vi "REPL_Comm.vi"(8 "REPL Name":string="Robot  REPL", 9 "CodeRef":refnum<vi>, 11 "Microprocessor in":T2) -> (3 "Microprocessor out":T2)   [LabVIEW 2016]
uses:
  uPythonX/uPythonX.xctl
  ColorText/Code.xctl
  <vilib>/Utility/miscctls.llb/LVPointTypeDef.ctl
panel:
  out "mouse down?":bool
  in  "VISA":refnum<visa-resource-name>
  out "Old Code":string
  in  "Files":u16(ring) items=["README.txt", "Screen.py", "boot.py", "fwupdate.mpy", "pybcdc.inf", "main.py"]
  in  "Ctrls":T1(ring)
  in  "HelpCode":string
  in  "Stop Script":bool
  in  "Pause":bool
  in  "Help Button":bool
  in  "New":bool
  in  "Delete":bool
  in  "refresh":bool
  in  "Code":string(xcontrol)="import utime\n\nfor i in range(5):\n     led.value(0)\n     utime.sleep_ms(1000)\n     led.value(1)\n     utime.sleep_ms(1000)\n\n\n\nprint('hi')"
  out "Script":string
  in  "Copy":bool
  out "String":string
  in  "Clear":bool
  out "Origin":T3
  in  "Ctrl D":bool
  in  "Ctrl C":bool
  in  "Run DIrect":bool
  in  "Run":bool
  out "Console":string
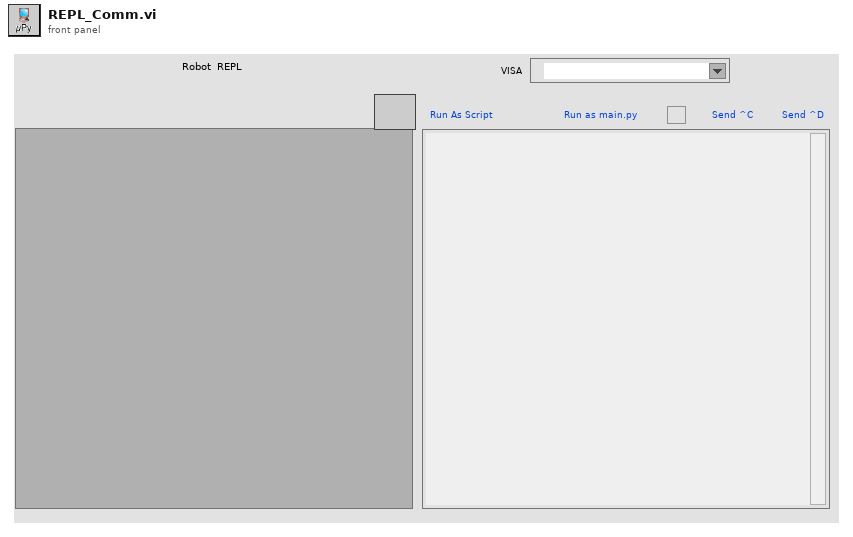
[diagram p1: front panel]
types:
  T1 = enum16{"File Control", "Save to PC", "Read from PC", "Save to MP as..."}
  T2 = cluster{"VISA Refnum in":refnum<visa-resource-name>, "Python Code":string}
  T3 = typedef "LVPointTypeDef.ctl" = cluster{"Horizontal":i16, "Vertical":i16}
  T4 = cluster{"VISA out":refnum<visa-resource-name>, "Code":string}
  T5 = typedef "eventvkey.ctl" = enum16{"ASCII", "Enter", "Return", "Shift", "Ctrl", "Alt", "Cmd", "Opt", "Caps", "NumLock", "Clear", "Break", "Up", "Down", "Left", "Right", "Insert", "Delete", "Home", "End", "PageUp", "PageDown", "Escape", "Help", "Pause", "ScrollLock", "F1", "F2", "F3", "F4", "F5", "F6", "F7", "F8", "F9", "F10", "F11", "F12", "F13", "F14", "F15", "F16", "F17", "F18", "F19", "F20", "F21", "F22", "F23", "F24", "Play", "VolumeUp", "VolumeDown", "Mute", "Two Byte Char"}
  T6 = cluster{"Shift":bool, "Ctrl":bool, "Alt":bool, "Cmd":bool, "Opt":bool}
  T7 = cluster{"Char":i16, "VKey":T5, "ScanCode":i16, "Mods":cluster{"Num Pad":bool, "Menu Key":bool}, "PlatMods":cluster{"Shift":bool, "Ctrl":bool, "Alt":bool, "Cmd":bool, "Opt":bool}, "FocusObj":refnum<vi>}
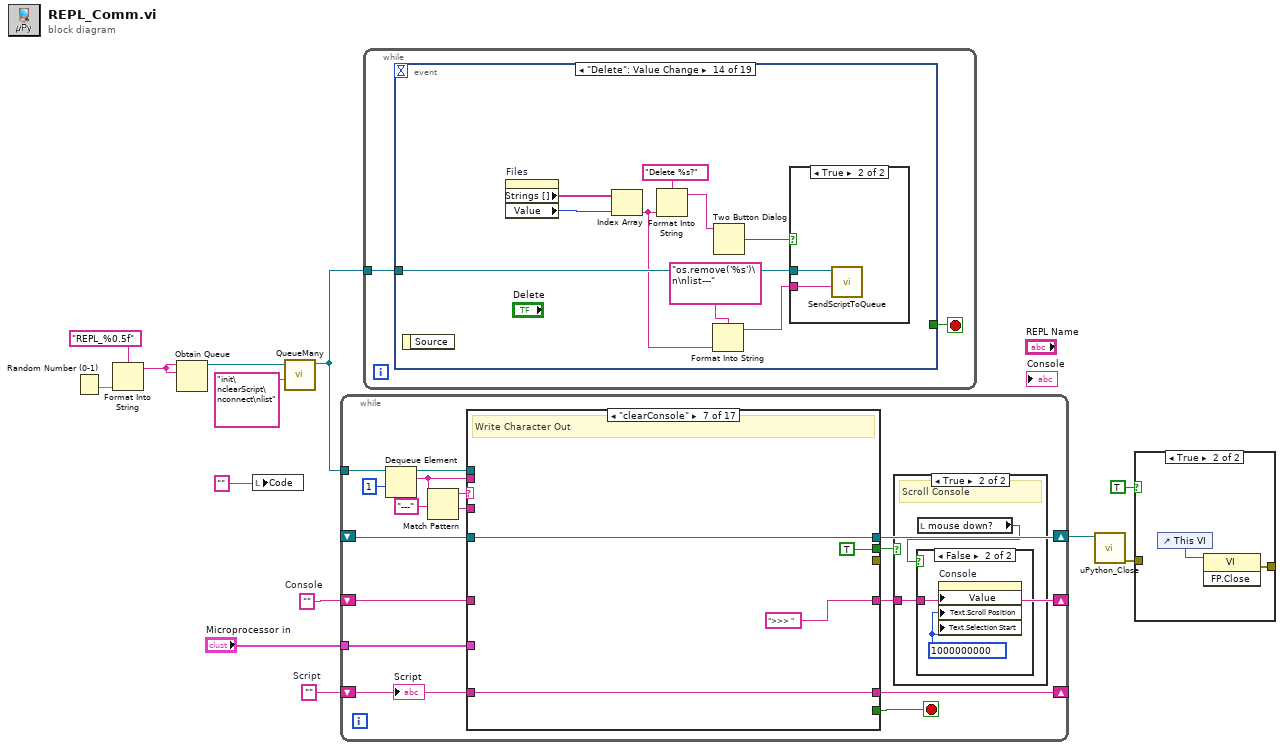
[diagram p0: block diagram]
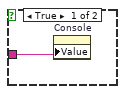
[diagram p4: hidden frame]
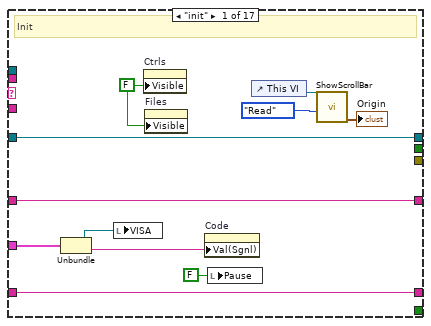
[diagram p5: hidden frame]
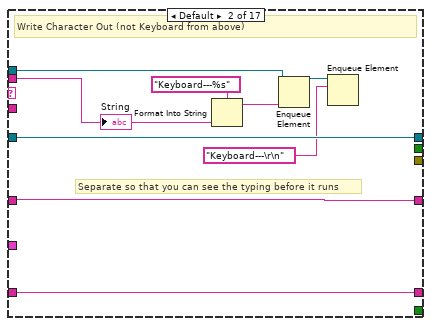
[diagram p6: hidden frame]
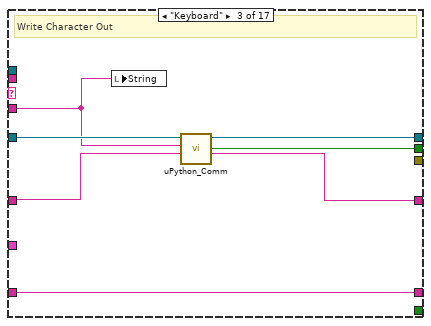
[diagram p7: hidden frame]
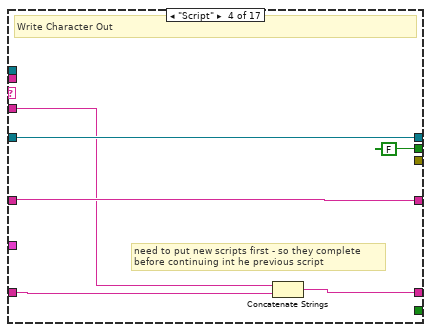
[diagram p8: hidden frame]
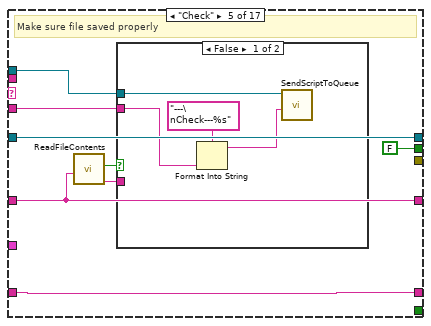
[diagram p9: hidden frame]
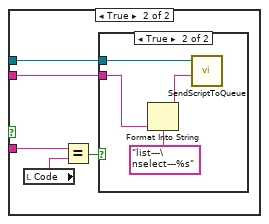
[diagram p10: hidden frame]
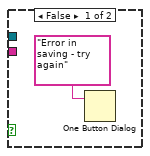
[diagram p11: hidden frame]
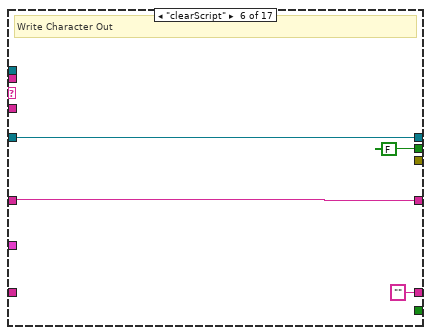
[diagram p12: hidden frame]
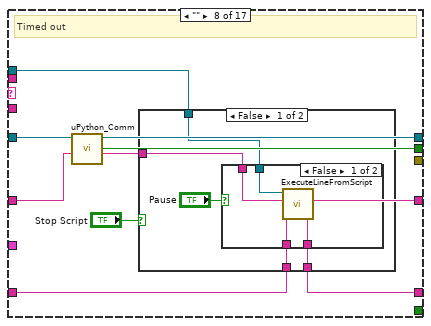
[diagram p13: hidden frame]
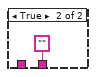
[diagram p15: hidden frame]
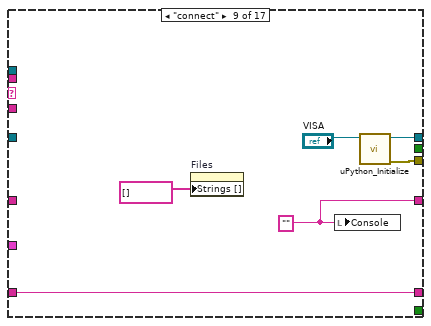
[diagram p16: hidden frame]
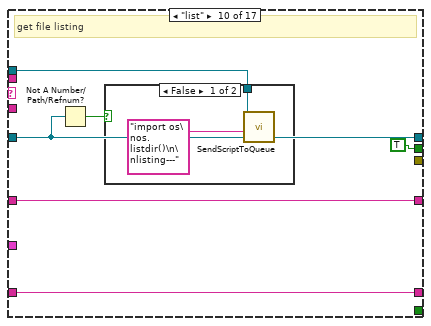
[diagram p17: hidden frame]
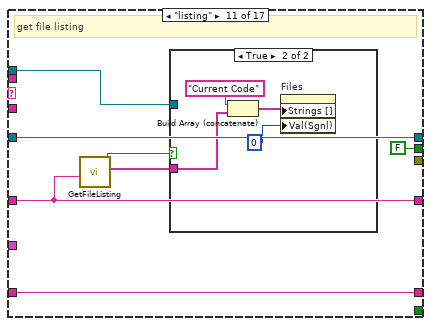
[diagram p19: hidden frame]
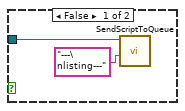
[diagram p20: hidden frame]
diagram:
  w8 = ""  # Script
  w9 = ""  # Console
  n1 = Random Number (0-1)() -> (number: 0 to 1=w2:dbl)
  n2 = Format Into String(format string="REPL_%0.5f" ("name (unnamed)"), w2) -> (resulting string=w1:string)  [unwired: 2 in, 1 out]
  n3 = Obtain Queue(name (unnamed)=w1, element data type=w1) -> (queue out=w13:refnum<queue>)  [unwired: 3 in, 2 out]
  n4 = local write "Code"("" ("Code")) -> ()
  n5 = call "QueueMany.vi"("Playlist"="init\nclearScript\nconnect\nlist" ("element"), "Queue in"=w13) -> ("Queue out"=w12:refnum<queue>)  [unwired: 9 in]
  n6 = while {
    tunnel: w12 -> [w29]
    shift-right: [w19] -> w10
    shift-left: _ -> [w27]
    shift-right: [w18] -> _
    shift-left: w9 -> [w20]
    shift-right: [w16] -> _
    shift-left: w8 -> [w15]
    tunnel: "Microprocessor in" -> [w14]
    stop <- w28 stop-if-true
    n7 = Dequeue Element(queue=w29, timeout in ms (-1)=1) -> (queue out=w25:refnum<queue>, element=w21:string)  [unwired: 1 in, 2 out]
    n8 = Match Pattern(string=w21, regular expression="---") -> (before substring=w23:string, after substring=w22:string)  [unwired: 1 in, 2 out]
    n9 = case shown="\"clearConsole\"" w23 {
      tunnel: [_ _ _ _ _ _ _ _ _ _ _ _ _ _ _ _ TRUE] -> w28
      tunnel: w27 -> [w45 w53 w60 w67 w75 w93 w97 w103 _ w125 w135 w148 w153 w173 w179 w185 w196]
      tunnel: w25 -> [_ w46 _ _ w71 _ _ w106 _ w127 w132 w145 _ _ _ _ _]
      tunnel: w22 -> [_ _ w55 w62 w68 _ _ _ _ _ _ _ _ w174 _ _ _]
      tunnel: w21 -> [_ w48 _ _ _ _ _ _ _ _ _ _ _ _ _ _ _]
      tunnel: [w45 w53 w58 w67 w75 w93 w97 w100 w123 w125 w135 w148 w161 w173 w179 w185 w196] -> w19
      tunnel: w20 -> [w44 w52 w59 w66 w70 w92 _ w102 _ w126 w134 w147 w156 w172 w182 w187 w197]
      tunnel: [w44 w52 w57 w66 w70 w92 ">>> " ("Console") w101 w121 w126 w134 w147 w159 w172 w182 w187 w197] -> w18
      tunnel: [_ _ _ _ _ _ _ _ w122 _ _ _ w158 _ _ _ _] -> _
      tunnel: [_ _ w56 FALSE ("Update?") FALSE ("Update?") FALSE ("Update?") TRUE ("Update?") w99 _ TRUE ("Update?") FALSE ("Update?") _ _ _ _ _ _] -> w17
      tunnel: [w42 w54 w61 w64 w73 "" ("Script") w95 w105 w119 w128 w136 w150 w167 w171 w181 w186 w194] -> w16
      tunnel: w15 -> [w42 w54 w61 w63 w73 _ w95 w104 w119 w128 w136 w150 w167 w171 w181 w186 w194]
      tunnel: w14 -> [w41 _ _ _ _ _ _ _ _ _ _ _ _ _ _ _ w192]
      frame "init" {
        w38 = FALSE ("Visible")
        # "Init"
        n10 = Unbundle(w41) -> ("VISA Refnum in"=w43:refnum<visa-resource-name>, "Python Code"=w40:string)
        n11 = local write "VISA"(w43) -> ()
        n12 = property on="Ctrls" class="Enum (strict)"("Visible"=w38) -> ()  [unwired: 2 in, 2 out]
        n13 = property on="Files" class="Ring (strict)"("Visible"=w38) -> ()  [unwired: 2 in, 2 out]
        n14 = property on="Code" class="Code (strict)"("Val(Sgnl)"=w40) -> ()  [unwired: 2 in, 2 out]
        n15 = local write "Pause"(FALSE ("Pause")) -> ()
        n16 = control-ref of="This VI"() -> (w37:refnum<vi>)
        n17 = call "ShowScrollBar.vi"("Task"=enum16{"Read", "Change", "Reset"}."Read", "VI in"=w37) -> ("Origin"=→"Origin":T3)  [unwired: 9 in]
      }
      frame Default {
        # "Separate so that you can see the typing before it runs"
        # "Write Character Out (not Keyboard from above)"
        n18 = Format Into String(format string="Keyboard---%s", w48) -> (resulting string=w50:string)  [unwired: 2 in, 1 out]
        n19 = Enqueue Element(queue=w46, element=w50) -> (queue out=w49:refnum<queue>)  [unwired: 2 in, 2 out]
        n20 = Enqueue Element(queue=w49, element="Keyboard---\r\n" ("regular expression")) -> ()  [unwired: 2 in, 3 out]
        "String" <- w48
      }
      frame "Keyboard" {
        # "Write Character Out"
        n21 = local write "String"(w55) -> ()
        n22 = call "uPython_Comm.vi"("Console In"=w59, "Script"=w55, "VISA Refnum in"=w60) -> ("Console Out"=w57:string, "VISA out"=w58:refnum<visa-resource-name>, "Update?"=w56:bool)  [unwired: 4 in, 2 out]
      }
      frame "Script" {
        # "need to put new scripts first - so they complete\nbefore continuing int he previous script"
        # "Write Character Out"
        n23 = Concatenate Strings(w62, w63) -> (w64:string)
      }
      frame "Check" {
        # "Make sure file saved properly"
        n24 = call "ReadFileContents.vi"("Console"=w70) -> ("File Contents"=w69:string, "Success?"=w72:bool)  [unwired: 9 in]
        n25 = case shown="False" w72 {
          tunnel: w71 -> [w79 w80]
          tunnel: w69 -> [_ w83]
          tunnel: w68 -> [w77 w82]
          frame False {
            n26 = Format Into String(format string="---\nCheck---%s" ("String"), w77) -> (resulting string=w76:string)  [unwired: 2 in, 1 out]
            n27 = call "SendScriptToQueue.vi"("String"=w76, "Queue in"=w79) -> ()  [unwired: 10 in]
          }
          frame True {
            n28 = local read "Code"() -> (w84:string)
            n29 = Equal?(x=w83, y=w84) -> (x = y?=w81:bool)
            n30 = case shown="True" w81 {
              tunnel: w82 -> [_ w88]
              tunnel: w80 -> [_ w87]
              frame False {
                n31 = One Button Dialog(message="Error in saving - try again" ("Code")) -> ()  [unwired: 1 in, 1 out]
              }
              frame True {
                n32 = Format Into String(format string="list---\nselect---%s" ("element"), w88) -> (resulting string=w86:string)  [unwired: 2 in, 1 out]
                n33 = call "SendScriptToQueue.vi"("String"=w86, "Queue in"=w87) -> ()  [unwired: 10 in]
              }
            }
          }
        }
      }
      frame "clearScript" {
        # "Write Character Out"
      }
      frame "clearConsole" {
        # "Write Character Out"
      }
      frame "" {
        # "Timed out"
        n34 = call "uPython_Comm.vi"("Console In"=w102, "VISA Refnum in"=w103) -> ("Console Out"=w101:string, "VISA out"=w100:refnum<visa-resource-name>, "Update?"=w99:bool)  [unwired: 5 in, 2 out]
        n35 = case shown="False" "Stop Script" {
          tunnel: w106 -> [w111 _]
          tunnel: [w110 "" ("Script")] -> w105
          tunnel: w104 -> [w109 _]
          tunnel: w101 -> [w108 _]
          frame False {
            n36 = case shown="False" "Pause" {
              tunnel: w111 -> [w115 _]
              tunnel: [w114 w116] -> w110
              tunnel: w109 -> [w113 w116]
              tunnel: w108 -> [w112 _]
              frame False {
                n37 = call "ExecuteLineFromScript.vi"("Script in"=w113, "Console"=w112, "Queue in"=w115) -> ("Script out"=w114:string)  [unwired: 8 in]
              }
              frame True {
              }
            }
          }
          frame True {
          }
        }
      }
      frame "connect" {
        w121 = "" ("element")
        n38 = property on="Files" class="Ring (strict)"("Strings []"=string[] [] ("Item Names")) -> ()  [unwired: 2 in, 2 out]
        n39 = local write "Console"(w121) -> ()
        n40 = call "uPython_Initialize.vi"("VISA Refnum in"="VISA") -> ("error out"=w122:errorcluster, "VISA Refnum out"=w123:refnum<visa-resource-name>)  [unwired: 9 in]
      }
      frame "list" {
        # "get file listing"
        n41 = Not A Number/Path/Refnum?(number/path/refnum=w125) -> (NaN/Path/Refnum?=w124:bool)
        n42 = case shown="False" w124 {
          tunnel: w127 -> [w131 _]
          frame False {
            n43 = call "SendScriptToQueue.vi"("String"="import os\nos.listdir()\n\nlisting---" ("element"), "Queue in"=w131) -> ()  [unwired: 10 in]
          }
          frame True {
          }
        }
      }
      frame "listing" {
        # "get file listing"
        n44 = call "GetFileListing.vi"("Console In"=w134) -> ("Files"=w138:string[], "Success?"=w133:bool)  [unwired: 9 in]
        n45 = case shown="True" w133 {
          tunnel: w138 -> [_ w144]
          tunnel: w132 -> [w139 _]
          frame False {
            n46 = call "SendScriptToQueue.vi"("String"="---\nlisting---", "Queue in"=w139) -> ()  [unwired: 10 in]
          }
          frame True {
            n47 = Build Array (concatenate)("Current Code", w144) -> (w143:string[])
            n48 = property on="Files" class="Ring (strict)"("Strings []"=w143, "Val(Sgnl)"=0) -> ()  [unwired: 2 in, 2 out]
          }
        }
      }
      frame "read" {
        n49 = call "ReadFileContents.vi"("Console"=w147) -> ("File Contents"=w149:string, "Success?"=w146:bool)  [unwired: 9 in]
        n50 = local write "Code"(w149) -> ()
        n51 = case shown="False" w146 {
          tunnel: w145 -> [w152 _]
          frame False {
            n52 = call "SendScriptToQueue.vi"("String"="---\nread---", "Queue in"=w152) -> ()  [unwired: 10 in]
          }
          frame True {
          }
        }
      }
      frame "run" {
        w157 = "\u0003"  # Ctrl C
        w164 = "\u0004"  # Ctrl D
        # "run on main.py"
        n53 = call "uPython_Comm.vi"("Console In"=w156, "Script"=w157, "VISA Refnum in"=w153) -> ("error out"=w155:errorcluster, "VISA out"=w154:refnum<visa-resource-name>)  [unwired: 4 in, 3 out]
        n54 = local read "Code"() -> (w160:string)
        n55 = call "SavePyFile.vi"("Name"="main.py", "error in"=w155, "Python Code"=w160, "VISA in"=w154) -> ("error out"=w165:errorcluster, "Reply"=w163:string, "VISA out"=w166:refnum<visa-resource-name>)  [unwired: 5 in]
        n56 = call "uPython_Comm.vi"("error in (no error)"=w165, "Console In"=w163, "Script"=w164, "VISA Refnum in"=w166) -> ("error out"=w158:errorcluster, "Console Out"=w159:string, "VISA out"=w161:refnum<visa-resource-name>)  [unwired: 3 in, 2 out]
      }
      frame "select" {
        n57 = property on="Files" class="Ring (strict)"() -> ("Strings []"=w168:string[])  [unwired: 2 in, 2 out]
        n58 = call <vilib>:"Trim Whitespace.vi"("string"=w174) -> ("trimmed string"=w170:string)  [unwired: 1 in]
        n59 = Search 1D Array(1D array=w168, element=w170) -> (index of element=w169:i32)  [unwired: 1 in]
        n60 = case shown="Default" w169 {
          selector: w169 -> [_ w175]
          frame -1 {
          }
          frame Default {
            n61 = property on="Files" class="Ring (strict)"("Val(Sgnl)"=w175) -> ()  [unwired: 2 in, 2 out]
          }
        }
      }
      frame "help" {
        n62 = local read "Code"() -> (w180:string)
        n63 = control-ref of="HelpCode"() -> (w176:refnum<vi>)
        n64 = Bundle("VISA out"=w179, "Code"=w180) -> (w178:T4)  [unwired: 1 in]
        n65 = call "OpenHelp.vi"("Code Ref"=w176, "Microprocessor in"=w178, "Dialog"=enum16{"REPL", "Help"}."Help") -> ()  [unwired: 9 in]
      }
      frame "update" {
        n66 = local read "Code"() -> (w183:string)
        n67 = property class="Str"(reference="CodeRef", "Val(Sgnl)"=w183) -> ()  [unwired: 1 in, 2 out]
      }
      frame "done" {
        w191 = FALSE ("Visible")
        n68 = local read "Code"() -> (w193:string)
        n69 = property on="Ctrls" class="Enum (strict)"("Visible"=w191) -> ()  [unwired: 2 in, 2 out]
        n70 = Bundle(cluster=w192, "VISA Refnum in"=w196, "Python Code"=w193) -> (→"Microprocessor out":T2)
        n71 = property on="Files" class="Ring (strict)"("Visible"=w191) -> ()  [unwired: 2 in, 2 out]
        n72 = control-ref of="This VI"() -> (w189:refnum<vi>)
        n73 = local read "Origin"() -> (w190:T3)
        n74 = call "ShowScrollBar.vi"("Origin in"=w190, "Task"=enum16{"Read", "Change", "Reset"}."Reset", "VI in"=w189) -> ()  [unwired: 8 in, 1 out]
      }
    }
    n75 = case shown="True" w17 {
      tunnel: w18 -> [_ w31]
      frame False {
      }
      frame True {
        # "Scroll Console"
        n76 = local read "mouse down?"() -> (w30:bool)
        n77 = case shown="False" w30 {
          tunnel: w31 -> [w32 w33]
          frame True {
            n78 = property on="Console" class="Str"("Value"=w32) -> ()  [unwired: 2 in, 2 out]
          }
          frame False {
            w34 = u32 1000000000 ("Text.Selection:Start")
            n79 = property on="Console" class="Str"("Value"=w33, "Text.Scroll Position"=w34, "Text.Selection Start"=w34) -> ()  [unwired: 2 in, 2 out]
          }
        }
      }
    }
    "Script" <- w15
  }
  n80 = while {
    tunnel: w12 -> [w199]
    stop <- w200 stop-if-true
    n81 = event shown="[13] \"Delete\": Value Change" {
      selector: _ -> [_ _ _ _ _ _ _ _ _ _ _ _ _ _ _ _ _ _ _]
      dyn-events: _ -> [_ _ _ _ _ _ _ _ _ _ _ _ _ _ _ _ _ _ _]
      timeout: _ -> [_ _ _ _ _ _ _ _ _ _ _ _ _ _ _ _ _ _ _]
      tunnel: w199 -> [w202 _ _ _ w212 w225 w249 w258 w262 w285 w289 w291 w292 w299 w306 w307 w309 _ w312]
      tunnel: [_ _ _ _ TRUE ("Discard?") _ _ _ _ _ _ _ _ _ _ _ _ _ _] -> w200
      event "Copy": Value Change {
        n82 = event-data() -> ()  [unwired: 1 in, 1 out]
        n83 = call "QueueMany.vi"("Playlist"="update" ("element"), "Queue in"=w202) -> ()  [unwired: 9 in, 1 out]
      }
      event Timeout {
        n84 = event-data() -> ()  [unwired: 1 in, 3 out]
      }
      event Mouse Down {
        n85 = event-data() -> ()  [unwired: 1 in, 8 out]
        "mouse down?" <- TRUE ("mouse down?")
      }
      event Mouse Leave; Mouse Up {
        n86 = event-data() -> ()  [unwired: 1 in, 4 out]
        n87 = local write "mouse down?"(FALSE ("mouse down?")) -> ()
      }
      event Panel Close? {
        n88 = event-data() -> ()  [unwired: 1 in, 1 out]
        n89 = local read "Microprocessor in"() -> (w208:T2)
        n90 = local read "Code"() -> (w207:string)
        n91 = Unbundle By Name(w208) -> ("Python Code"=w206:string)
        n92 = Not Equal?(x=w206, y=w207) -> (x != y?=w205:bool)
        n93 = case shown="True" w205 {
          tunnel: ["done" ("element") w214] -> w209
          frame False {
          }
          frame True {
            n94 = Two Button Dialog(message="Do you want to update your program?", 1:"Revert" ("F button name (\"Cancel\")"), 2:"Update" ("T button name (\"OK\")")) -> (T button?=w217:bool)
            n95 = Select(t="update\ndone" ("element"), s=w217, f="done" ("element")) -> (s? t:f=w214:string)
          }
        }
        n96 = call "QueueMany.vi"("Playlist"=w209, "Queue in"=w212) -> ()  [unwired: 9 in, 1 out]
        n97 = event-data("Discard?"=TRUE) -> ()  [unwired: 1 in, 1 out]
      }
      event Key Down {
        n98 = event-data() -> ("Char"=w229:i16, "VKey"=w221:T5, "ScanCode"=w228:i16, "Mods"=w227:cluster{"Num Pad":bool, "Menu Key":bool}, "PlatMods"=w226:T6, "FocusObj"=w224:refnum<vi>)  [unwired: 1 in]
        n99 = case shown="\"F4\"" w221 {
          frame "ASCII", Default {
          }
          frame "F4" {
            n100 = control-ref of="This VI"() -> (w232:refnum<vi>)
            n101 = property on="Ctrls" class="Enum (strict)"() -> ("Visible"=w233:bool)  [unwired: 2 in, 2 out]
            n102 = case shown="False" w233 {
              tunnel: [FALSE ("Visible") TRUE ("Visible")] -> w231
              tunnel: w232 -> [w236 w240]
              frame True {
                n103 = local read "Origin"() -> (w234:T3)
                n104 = call "ShowScrollBar.vi"("Origin in"=w234, "Task"=enum16{"Read", "Change", "Reset"}."Reset", "VI in"=w236) -> ()  [unwired: 8 in, 1 out]
              }
              frame False {
                n105 = local read "Origin"() -> (w238:T3)
                n106 = call "ShowScrollBar.vi"("Origin in"=w238, "Task"=enum16{"Read", "Change", "Reset"}."Change", "VI in"=w240) -> ()  [unwired: 8 in, 1 out]
              }
            }
            n107 = property on="Ctrls" class="Enum (strict)"("Visible"=w231) -> ()  [unwired: 2 in, 2 out]
            n108 = property on="Files" class="Ring (strict)"("Visible"=w231) -> ()  [unwired: 2 in, 2 out]
          }
        }
        n109 = Bundle("Char"=w229, "VKey"=w221, "ScanCode"=w228, "Mods"=w227, "PlatMods"=w226, "FocusObj"=w224) -> (w230:T7)  [unwired: 1 in]
        n110 = control-ref of="Code"() -> (w222:refnum<vi>)
        n111 = Not Equal?(x=w224, y=w222) -> (x != y?=w223:bool)
        n112 = case shown="True" w223 {
          tunnel: w230 -> [_ w244]
          tunnel: w225 -> [_ w243]
          frame False {
          }
          frame True {
            n113 = call "TranslateTyping.vi"("Cluster"=w244) -> ("string"=w242:string)  [unwired: 10 in]
            n114 = call "QueueMany.vi"("Playlist"=w242, "Queue in"=w243) -> ()  [unwired: 9 in, 1 out]
          }
        }
      }
      event "Files": Value Change {
        n115 = event-data() -> ("OldVal"=w245:u16)  [unwired: 1 in]
        n116 = property on="Files" class="Ring (strict)"() -> ("Strings []"=w247:string[])  [unwired: 2 in, 2 out]
        n117 = Index Array(array=w247, index="Files") -> (element=w246:string)
        n118 = case shown="Default" w246 {
          selector: w246 -> [_ w252]
          tunnel: w249 -> [_ w254]
          tunnel: w245 -> [_ w251]
          frame "Current Code" {
            n119 = local read "Old Code"() -> (w250:string)
            n120 = local write "Code"(w250) -> ()
          }
          frame Default {
            n121 = case shown="0" w251 {
              frame 0 {
                n122 = local read "Code"() -> (→"Old Code":string)
              }
              frame Default {
              }
            }
            n123 = Format Into String(format string="Script---file = open('%s','rb')\ntext = file.read()\nfile.close()\n\ntext\nread---" ("write buffer"), w252) -> (resulting string=w253:string)  [unwired: 2 in, 1 out]
            n124 = call "SendScriptToQueue.vi"("String"=w253, "Queue in"=w254) -> ()  [unwired: 10 in]
          }
        }
      }
      event "refresh": Value Change {
        n125 = event-data() -> ()  [unwired: 1 in, 1 out]
        n126 = call "QueueMany.vi"("Playlist"="list" ("element"), "Queue in"=w258) -> ()  [unwired: 9 in, 1 out]
      }
      event "Ctrls": Value Change {
        n127 = event-data() -> ()  [unwired: 1 in, 1 out]
        n128 = case shown="\"Save to PC\"" "Ctrls" {
          tunnel: w262 -> [_ _ w273 _]
          tunnel: [w263 w264 w272 w275] -> w260
          tunnel: T1."File Control" ("Ctrls") -> [w263 w264 w272 w275]
          frame Default {
            # "Default"
          }
          frame "Read from PC" {
            # "Open PC file"
            n129 = call "File Dialog"("prompt"="Find File") -> ("selected path"=w268:path, "cancelled"=w267:bool, "error out"=w265:errorcluster)  [unwired: 11 in, 1 out]
            n130 = case shown="False" w267 {
              tunnel: w268 -> [w271 _]
              tunnel: w265 -> [_ _]
              frame False {
                n131 = Read from Text File(file (use dialog)=w271, count=-1) -> (text=w270:string)  [unwired: 2 in, 3 out]
                n132 = local write "Code"(w270) -> ()
              }
              frame True {
              }
            }
          }
          frame "Save to MP as..." {
            # "Save As... on MP"
            n133 = local read "Code"() -> (w274:string)
            n134 = call "SaveOnMP.vi"("Contents"=w274, "Queue in"=w273) -> ()  [unwired: 10 in]
          }
          frame "Save to PC" {
            # "Save to PC"
            n135 = call "File Dialog2"("prompt"="Select File") -> ("selected path"=w279:path, "cancelled"=w278:bool, "error out"=w276:errorcluster)  [unwired: 11 in, 1 out]
            n136 = case shown="False" w278 {
              tunnel: w279 -> [w280 _]
              tunnel: w276 -> [_ _]
              frame False {
                n137 = local read "Code"() -> (w281:string)
                n138 = Write to Text File(file (use dialog)=w280, text=w281) -> ()  [unwired: 2 in, 3 out]
              }
              frame True {
              }
            }
          }
        }
        n139 = local write "Ctrls"(w260) -> ()
      }
      event "Ctrl C": Value Change {
        w284 = "\u0003"  # Ctrl C
        n140 = event-data() -> ()  [unwired: 1 in, 1 out]
        n141 = call "QueueMany.vi"("Playlist"=w284, "Queue in"=w285) -> ("Queue out"=w283:refnum<queue>)  [unwired: 9 in]
        n142 = call "QueueMany.vi"("Playlist"="clearScript" ("element"), "Queue in"=w283) -> ()  [unwired: 9 in, 1 out]
      }
      event "Ctrl D": Value Change {
        w288 = "\u0004"  # Ctrl D
        n143 = event-data() -> ()  [unwired: 1 in, 1 out]
        n144 = call "QueueMany.vi"("Playlist"=w288, "Queue in"=w289) -> ("Queue out"=w286:refnum<queue>)  [unwired: 9 in]
        n145 = call "QueueMany.vi"("Playlist"="clearScript" ("element"), "Queue in"=w286) -> ()  [unwired: 9 in, 1 out]
      }
      event "Run DIrect": Value Change {
        n146 = event-data() -> ()  [unwired: 1 in, 1 out]
        n147 = call "SendScriptToQueue.vi"("String"="Code", "Queue in"=w291) -> ()  [unwired: 10 in]
      }
      event "Run": Value Change {
        n148 = event-data() -> ()  [unwired: 1 in, 1 out]
        n149 = call "QueueMany.vi"("Playlist"="run" ("element"), "Queue in"=w292) -> ()  [unwired: 9 in, 1 out]
      }
      event "Delete": Value Change {
        n150 = event-data() -> ()  [unwired: 1 in, 1 out]
        n151 = property on="Files" class="Ring (strict)"() -> ("Strings []"=w295:string[], "Value"=w294:u16)  [unwired: 2 in, 2 out]
        n152 = Index Array(array=w295, index=w294) -> (element=w298:string)
        n153 = Format Into String(format string="Delete %s?", w298) -> (resulting string=w302:string)  [unwired: 2 in, 1 out]
        n154 = Format Into String(format string="os.remove('%s')\n\nlist---" ("element"), w298) -> (resulting string=w297:string)  [unwired: 2 in, 1 out]
        n155 = Two Button Dialog(message=w302) -> (T button?=w300:bool)  [unwired: 2 in]
        n156 = case shown="True" w300 {
          tunnel: w299 -> [_ w304]
          tunnel: w297 -> [_ w303]
          frame False {
          }
          frame True {
            n157 = call "SendScriptToQueue.vi"("String"=w303, "Queue in"=w304) -> ()  [unwired: 10 in]
          }
        }
      }
      event "New": Value Change {
        w305 = "# place code here" ("Contents")
        n158 = event-data() -> ()  [unwired: 1 in, 1 out]
        n159 = local write "Code"(w305) -> ()
        n160 = call "SaveOnMP.vi"("Contents"=w305, "Queue in"=w306) -> ()  [unwired: 10 in]
      }
      event "VISA": Value Change {
        n161 = event-data() -> ()  [unwired: 1 in, 1 out]
        n162 = call "QueueMany.vi"("Playlist"="connect\nlist" ("element"), "Queue in"=w307) -> ()  [unwired: 9 in, 1 out]
      }
      event "Help Button": Value Change {
        n163 = event-data() -> ()  [unwired: 1 in, 1 out]
        n164 = call "QueueMany.vi"("Playlist"="help" ("element"), "Queue in"=w309) -> ()  [unwired: 9 in, 1 out]
      }
      event "HelpCode": Value Change {
        n165 = event-data() -> ()  [unwired: 1 in, 1 out]
        n166 = property on="Code" class="Code (strict)"("Val(Sgnl)"="HelpCode") -> ()  [unwired: 2 in, 2 out]
      }
      event "Clear": Value Change {
        n167 = event-data() -> ()  [unwired: 1 in, 2 out]
        n168 = call "QueueMany.vi"("Playlist"="clearConsole" ("element"), "Queue in"=w312) -> ()  [unwired: 9 in, 1 out]
      }
    }
  }
  n169 = call "uPython_Close.vi"("VISA  in"=w10) -> ("error out"=w6:errorcluster)  [unwired: 9 in, 1 out]
  n170 = case shown="True" TRUE {
    tunnel: w6 -> [_ _]
    tunnel: [_ w314] -> _
    frame False {
    }
    frame True {
      n171 = control-ref of="This VI"() -> (w315:refnum<vi>)
      n172 = invoke class="VI" method="FP.Close"(reference=w315) -> (error out=w314:errorcluster)  [unwired: 2 in, 2 out]
    }
  }
